vi "1_2_back.vi"(11 "Formatted 1D String Array":string[](array[string])) -> (3 "Array":string[](array[string]))   [LabVIEW 2023, in "2023.lvlib"]
uses:
  2023.lvlib
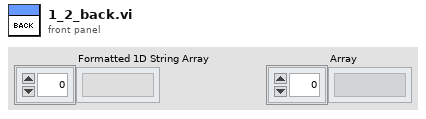
[diagram p1: front panel]
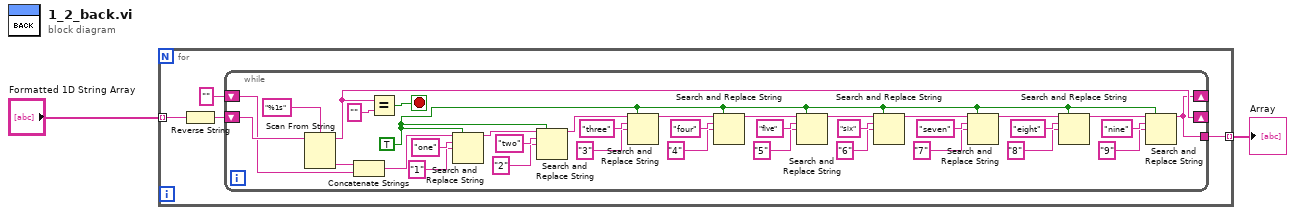
[diagram p0: block diagram]
diagram:
  n1 = for {
    tunnel: "Formatted 1D String Array" -> [w4] mode=indexing
    tunnel: [w6] -> w1 mode=indexing
    n2 = Reverse String(1:w4) -> (0:w3:string)
    n3 = while {
      tunnel: [w7] -> w6
      shift-right: [w10] -> _
      shift-left: w3 -> [w15]
      shift-right: [w7] -> _
      shift-left: "" -> [w12]
      stop <- w8 stop-if-true
      w18 = TRUE ("replace all? (F)")
      n4 = Scan From String(format string="%1s", input string=w15) -> (remaining string=w10:string, output 1=w13:string)  [unwired: 3 in, 2 out]
      n5 = Concatenate Strings(w13, w12) -> (w11:string)
      n6 = Equal?(x=w10, y="") -> (x = y?=w8:bool)
      n7 = Search and Replace String(replace all?=w18, input string=w11, search string="one", replace string="1" ("replace string (\"\")")) -> (result string=w40:string)  [unwired: 4 in, 3 out]
      n8 = Search and Replace String(replace all?=w18, input string=w40, search string="two", replace string="2" ("replace string (\"\")")) -> (result string=w37:string)  [unwired: 4 in, 3 out]
      n9 = Search and Replace String(replace all?=w18, input string=w37, search string="three", replace string="3" ("replace string (\"\")")) -> (result string=w36:string)  [unwired: 4 in, 3 out]
      n10 = Search and Replace String(replace all?=w18, input string=w36, search string="four", replace string="4" ("replace string (\"\")")) -> (result string=w35:string)  [unwired: 4 in, 3 out]
      n11 = Search and Replace String(replace all?=w18, input string=w35, search string="five", replace string="5" ("replace string (\"\")")) -> (result string=w34:string)  [unwired: 4 in, 3 out]
      n12 = Search and Replace String(replace all?=w18, input string=w34, search string="six", replace string="6" ("replace string (\"\")")) -> (result string=w33:string)  [unwired: 4 in, 3 out]
      n13 = Search and Replace String(replace all?=w18, input string=w33, search string="seven", replace string="7" ("replace string (\"\")")) -> (result string=w22:string)  [unwired: 4 in, 3 out]
      n14 = Search and Replace String(replace all?=w18, input string=w22, search string="eight", replace string="8" ("replace string (\"\")")) -> (result string=w19:string)  [unwired: 4 in, 3 out]
      n15 = Search and Replace String(replace all?=w18, input string=w19, search string="nine", replace string="9" ("replace string (\"\")")) -> (result string=w7:string)  [unwired: 4 in, 3 out]
    }
  }
  "Array" <- w1
